vi "Options Event.vi"(8 "error in (no error)":errorcluster, 11 "Shared Options in":refnum<class "Shared Options.lvclass">) -> (0 "error out":errorcluster, 2 "Options Event":refnum<user-event>, 3 "Shared Options out":refnum<class "Shared Options.lvclass">)   [LabVIEW 2020, in "AutoComplete.lvlib" / "Shared Options.lvclass"]
uses:
  Shared Options.lvclass
  Shared Options.lvclass/Shared Options.ctl
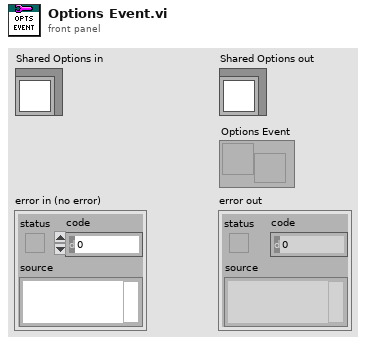
[diagram p1: front panel]
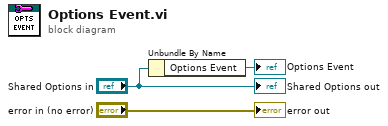
[diagram p0: block diagram]
diagram:
  n1 = Unbundle By Name("Shared Options in") -> ("Options Event"=→"Options Event":refnum<user-event>)
  "error out" <- "error in (no error)"
  "Shared Options out" <- "Shared Options in"
